vi "Instance RepCap.vi"(1 "Instance in":i32=1) -> (0 "Instance out":string)   [LabVIEW 2015, in "Rohde&Schwarz CMXP GPRF.lvlib"]
doc: "This VI performs a range check and formats the instance repcap string from a numeric input."
uses:
  <instrlib>/Rohde&Schwarz CMXP GPRF/Rohde&Schwarz CMXP GPRF.lvlib
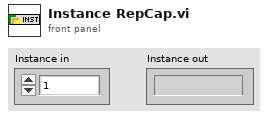
[diagram p1: front panel]
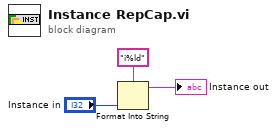
[diagram p0: block diagram]
diagram:
  n1 = Format Into String(format string="i%ld", "Instance in") -> (resulting string=→"Instance out":string)  [unwired: 2 in, 1 out]
